vi "Send Message.vi"(8 "error in":errorcluster, 11 "Message":T1) -> (0 "error out":errorcluster)   [LabVIEW 2016, in "Vision Server.lvclass"]
uses:
  Vision Server.lvclass
  typedef/Message Type.ctl
  Vision Server.lvclass/Vision Server.ctl
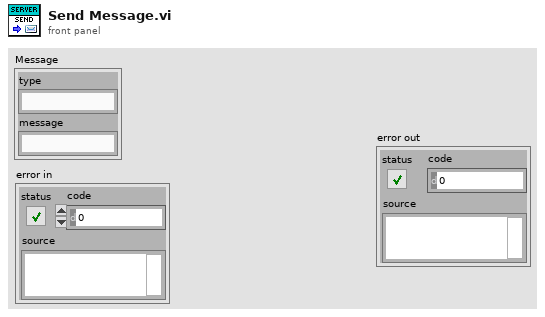
[diagram p1: front panel]
types:
  T1 = typedef "Vision Server.lvclass/Message Type.ctl" = cluster{"type":string, "message":string}
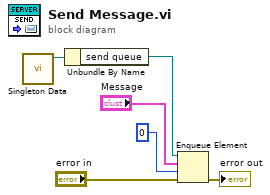
[diagram p0: block diagram]
diagram:
  n1 = call "Singleton Data.vi"() -> ("Vision Server Copy"=w6:refnum<class "Vision Server.lvclass">)  [unwired: 10 in, 1 out]
  n2 = Unbundle By Name(w6) -> ("send queue"=w5:refnum<queue>)
  n3 = Enqueue Element(queue=w5, element="Message", timeout in ms (-1)=0, error in (no error)="error in") -> (error out=→"error out":errorcluster)  [unwired: 2 out]
